vi "Data Display Switch.vi"(8 "error in":errorcluster, 10 "Path":string, 11 "Switch":T2(ring)) -> (0 "error out":errorcluster, 2 "Image Out":T1, 3 "Ascan":dbl[](array[numeric]))   [LabVIEW 2015, in "Utility VIs.lvlib"]
uses:
  Utility VIs.lvlib
  <vilib>/vision/Image Controls.llb/IMAQ Image.ctl
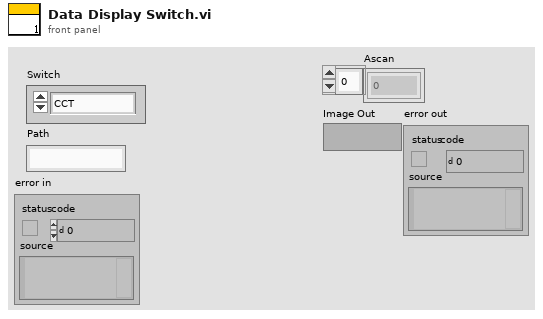
[diagram p1: front panel]
types:
  T1 = typedef "IMAQ Image.ctl" = refnum<image>
  T2 = enum16{"CCT", "ACD", "LT", "RT", "AL", "PD", "WTW", "K_flat", "K_steep", "K_AST"}
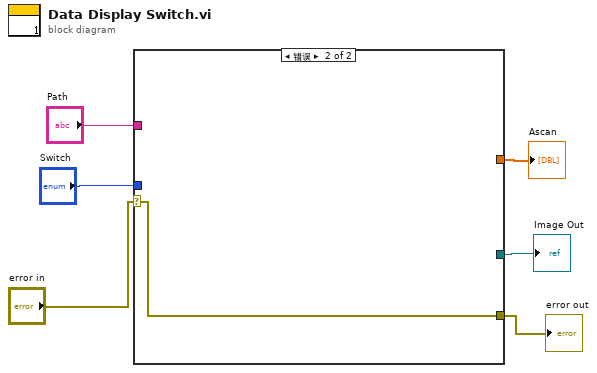
[diagram p0: block diagram]
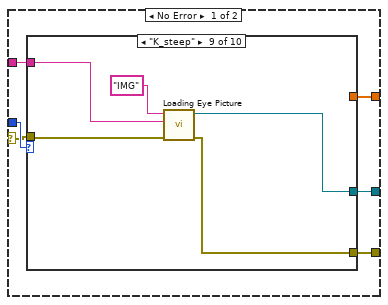
[diagram p2: hidden frame]
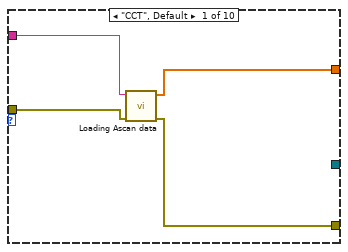
[diagram p3: hidden frame]
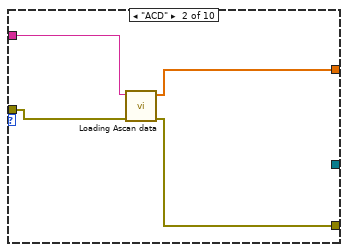
[diagram p4: hidden frame]
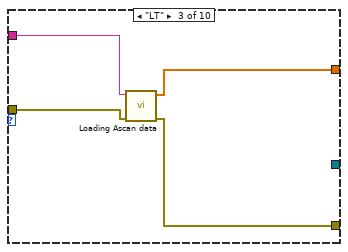
[diagram p5: hidden frame]
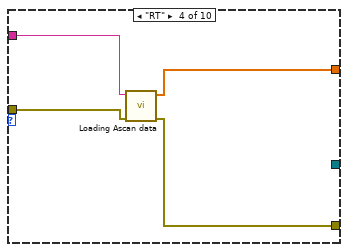
[diagram p6: hidden frame]
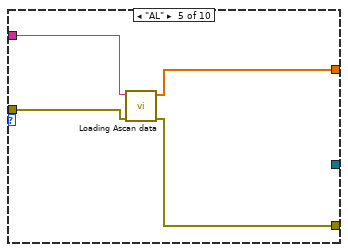
[diagram p7: hidden frame]
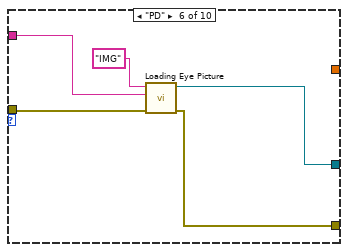
[diagram p8: hidden frame]
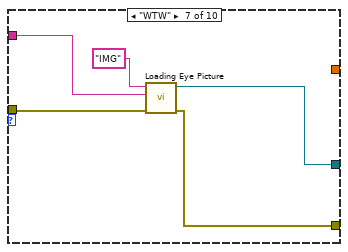
[diagram p9: hidden frame]
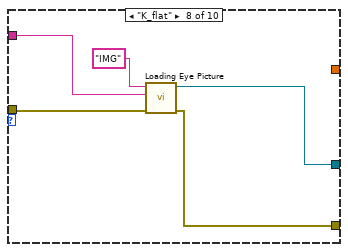
[diagram p10: hidden frame]
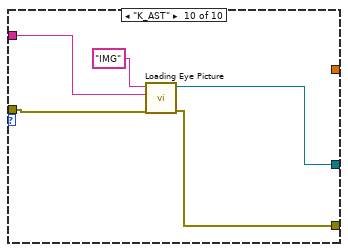
[diagram p11: hidden frame]
diagram:
  n1 = case shown="错误" "error in" {
    selector: "error in" -> [w8 w58]
    tunnel: "Switch" -> [w12 _]
    tunnel: "Path" -> [w11 _]
    tunnel: [w10 _] -> w4
    tunnel: [w9 _] -> w3
    tunnel: [w7 w58] -> w1
    frame No Error {
      n2 = case shown="\"K_steep\"" w12 {
        tunnel: w11 -> [w16 w20 w24 w28 w32 w37 w42 w47 w52 w57]
        tunnel: [w15 w19 w23 w27 w31 _ _ _ _ _] -> w10
        tunnel: [_ _ _ _ _ w35 w40 w45 w50 w55] -> w9
        tunnel: w8 -> [w14 w18 w22 w26 w30 w34 w38 w44 w49 w54]
        tunnel: [w13 w17 w21 w25 w29 w33 w39 w43 w48 w53] -> w7
        frame "CCT", Default {
          n3 = call "Loading Ascan data.vi"("error in (no error)"=w14, "名称或相对路径"=w16) -> ("error out"=w13:errorcluster, "first row"=w15:dbl[])  [unwired: 8 in]
        }
        frame "ACD" {
          n4 = call "Loading Ascan data.vi"("error in (no error)"=w18, "名称或相对路径"=w20) -> ("error out"=w17:errorcluster, "first row"=w19:dbl[])  [unwired: 8 in]
        }
        frame "LT" {
          n5 = call "Loading Ascan data.vi"("error in (no error)"=w22, "名称或相对路径"=w24) -> ("error out"=w21:errorcluster, "first row"=w23:dbl[])  [unwired: 8 in]
        }
        frame "RT" {
          n6 = call "Loading Ascan data.vi"("error in (no error)"=w26, "名称或相对路径"=w28) -> ("error out"=w25:errorcluster, "first row"=w27:dbl[])  [unwired: 8 in]
        }
        frame "AL" {
          n7 = call "Loading Ascan data.vi"("error in (no error)"=w30, "名称或相对路径"=w32) -> ("error out"=w29:errorcluster, "first row"=w31:dbl[])  [unwired: 8 in]
        }
        frame "PD" {
          n8 = call "Loading Eye Picture.vi"("error in (no error)"=w34, "名称或相对路径"=w37, "Image Name"="IMG") -> ("error out"=w33:errorcluster, "Image Out"=w35:T1)  [unwired: 7 in]
        }
        frame "WTW" {
          n9 = call "Loading Eye Picture.vi"("error in (no error)"=w38, "名称或相对路径"=w42, "Image Name"="IMG") -> ("error out"=w39:errorcluster, "Image Out"=w40:T1)  [unwired: 7 in]
        }
        frame "K_flat" {
          n10 = call "Loading Eye Picture.vi"("error in (no error)"=w44, "名称或相对路径"=w47, "Image Name"="IMG") -> ("error out"=w43:errorcluster, "Image Out"=w45:T1)  [unwired: 7 in]
        }
        frame "K_steep" {
          n11 = call "Loading Eye Picture.vi"("error in (no error)"=w49, "名称或相对路径"=w52, "Image Name"="IMG") -> ("error out"=w48:errorcluster, "Image Out"=w50:T1)  [unwired: 7 in]
        }
        frame "K_AST" {
          n12 = call "Loading Eye Picture.vi"("error in (no error)"=w54, "名称或相对路径"=w57, "Image Name"="IMG") -> ("error out"=w53:errorcluster, "Image Out"=w55:T1)  [unwired: 7 in]
        }
      }
    }
    frame Error {
    }
  }
  "Ascan" <- w4
  "Image Out" <- w3
  "error out" <- w1
